vi "Verify Min-Max Plot.vi"(1 "[user-specified font]":T1={"Font Name:"="Current Font", "Size"=36, "Strikeout?"=FALSE, "Italic?"=FALSE, "Underline?"=FALSE, "Outline?"=TRUE, "Shadow?"=TRUE, "Bold?"=TRUE}, 2 "desired font(Application)":T2(ring), 3 "Text To Draw":string) -> (0 "Min Max Plot":picture)   [LabVIEW 2010]
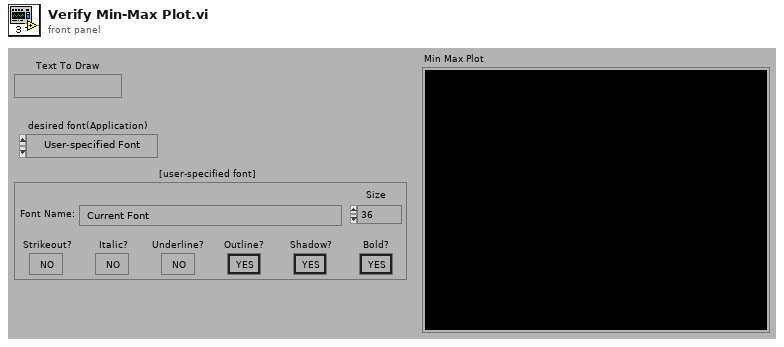
[diagram p1: front panel]
types:
  T1 = cluster{"Font Name:":string, "Size":i16, "Strikeout?":bool, "Italic?":bool, "Underline?":bool, "Outline?":bool, "Shadow?":bool, "Bold?":bool}
  T2 = enum16{"User-specified Font", "Application Font", "System Font", "Dialog Font"}
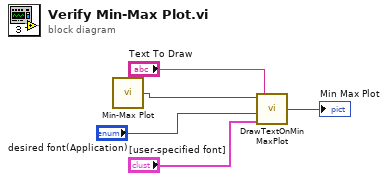
[diagram p0: block diagram]
diagram:
  n1 = call "Min-Max Plot.vi"() -> ("Min Max Plot"=w5:picture)  [unwired: 1 out]
  n2 = call "DrawTextOnMinMaxPlot.vi"("[user-specified font]"="[user-specified font]", "desired font(Application)"="desired font(Application)", "Text To Draw"="Text To Draw", "Min Max Plot In"=w5) -> ("Min Max Plot Out"=→"Min Max Plot":picture)
